vi "Turret_Aim.vi"(6 "Driver Right Thumb":bool, 7 "Left Trigger":dbl, 8 "Orange Limit Pressed":bool, 9 "Blue Limit Pressed":bool, 10 "Right Bumper":bool, 11 "Left Bumper":bool) -> ()   [LabVIEW 2020]
uses:
  <vilib>/Rock Robotics/WPI/ThirdParty/Phoenix-LabVIEW/Motor Controller/Controls/CTRE_Phoenix_MotorControl_ControlMode.ctl
  <vilib>/Rock Robotics/WPI/ThirdParty/Phoenix-LabVIEW/Motor Controller/Get/CTRE_Phoenix_MotorController_IntegratedSensorData_TalonFX.vi
  <vilib>/addons/control/pid/pid.llb/PID (DBL).vi
  <vilib>/Rock Robotics/Network Tables/NT Write Number.vi
  <vilib>/addons/control/pid/NI_PID_pid.lvlib
panel:
  in  "setpoint":dbl=1800.0 format="%#_13g"
  in  "Turret Home":T1={"proportional gain (Kc)"=0.005, "integral time (Ti, min)"=0.0, "derivative time (Td, min)"=2e-05} {"derivative time (Td, min)" format="%.6f"; "integral time (Ti, min)" format="%.3f"; "proportional gain (Kc)" format="%.3f"}
  out "Ty":dbl
  in  "PID gains 5":T1={"proportional gain (Kc)"=-0.015, "integral time (Ti, min)"=0.0, "derivative time (Td, min)"=2e-05} {"derivative time (Td, min)" format="%.6f"; "integral time (Ti, min)" format="%.3f"; "proportional gain (Kc)" format="%.3f"}
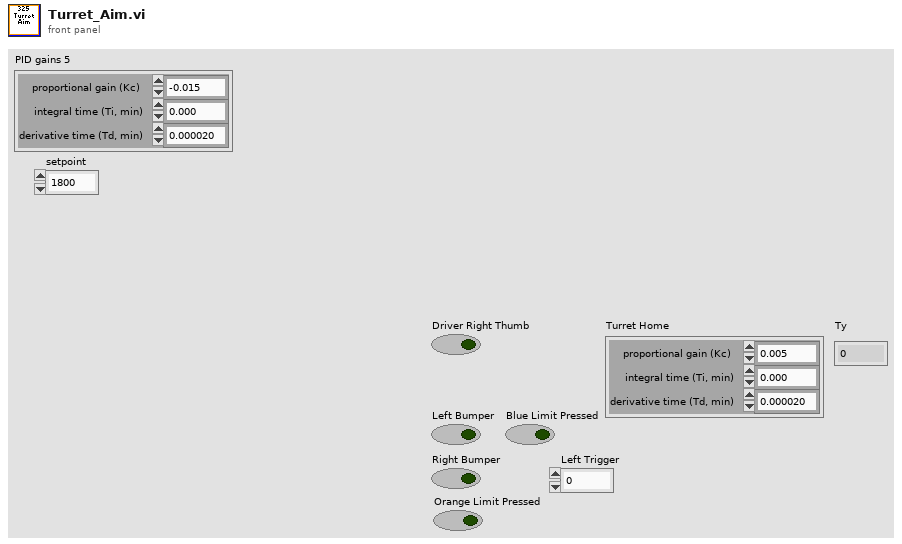
[diagram p1: front panel]
types:
  T1 = cluster{"proportional gain (Kc)":dbl, "integral time (Ti, min)":dbl, "derivative time (Td, min)":dbl}
  T2 = typedef "CTRE_Phoenix_MotorControl_ControlMode.ctl" = u16
  T3 = typedef "WPI_MotorControlDeviceRef.ctl" = cluster{"DeviceStatus":errorcluster, "Type":T4, "PWM":cluster{"PWM Channel":T5, "DeadBand":T6}, "CAN":cluster{"Device Number":u8, "SetOutput VI Ref":variant, "GetOutput VI Ref":variant, "Enable VI Ref":variant, "Disable VI Ref":variant, "Data":variant}, "Invert":bool, "DIO PWM":cluster{"PWM \"Enable\" Channel":T5, "DIOChannel":T7, "PWM Rate":dbl}}
  T4 = typedef "WPI_MotorControlType.ctl" = enum16{"PWM", "CAN", "DIO PWM"}
  T5 = typedef "FPGA_DIOPWMChannel.ctl" = enum8{"PWM 0", "PWM 1", "PWM 2", "PWM 3", "PWM 4", "PWM 5", "PWM 6", "PWM 7", "PWM 8", "PWM 9", "PWM MXP 0", "PWM MXP 1", "PWM MXP 2", "PWM MXP 3", "PWM MXP 4", "PWM MXP 5", "PWM MXP 6", "PWM MXP 7", "PWM MXP 8", "PWM MXP 9", "Invalid"}
  T6 = typedef "WPI_PWMDeadband.ctl" = cluster{"Name":string, "maxPositivePwm":i32, "minPositivePwm":i32, "centerPwm":i32, "maxNegativePwm":i32, "minNegativePwm":i32, "angularRange":u16}
  T7 = typedef "FPGA_DIOChannel.ctl" = enum8{"DIO 0", "DIO 1", "DIO 2", "DIO 3", "DIO 4", "DIO 5", "DIO 6", "DIO 7", "DIO 8", "DIO 9", "DIO MXP 0", "DIO MXP 1", "DIO MXP 2", "DIO MXP 3", "DIO MXP 4", "DIO MXP 5", "DIO MXP 6", "DIO MXP 7", "DIO MXP 8", "DIO MXP 9", "DIO MXP 10", "DIO MXP 11", "DIO MXP 12", "DIO MXP 13", "DIO MXP 14", "DIO MXP 15", "SPI Port CS1", "SPI Port CS2", "SPI Port CS3", "SPI Port MISO", "SPI Port MOSI", "Invalid"}
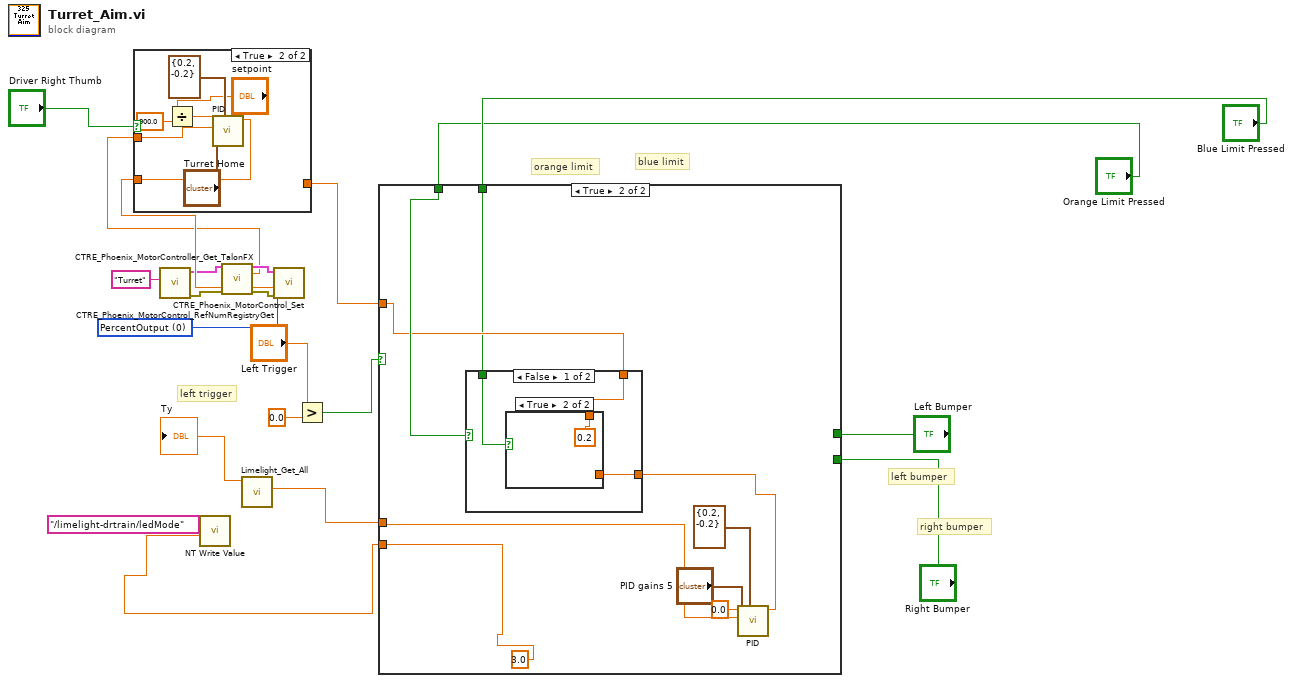
[diagram p0: block diagram]
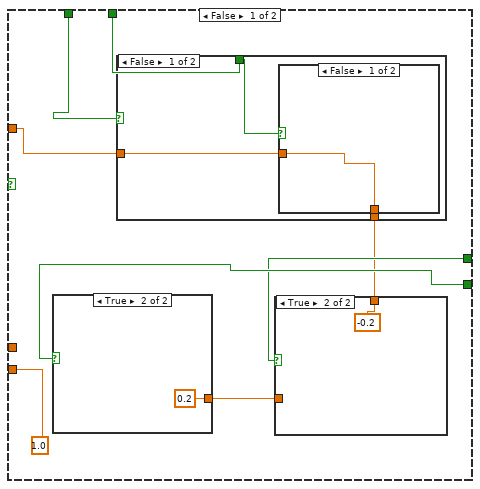
[diagram p3: hidden frame]
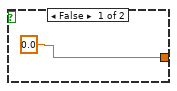
[diagram p5: hidden frame]
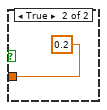
[diagram p6: hidden frame]
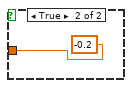
[diagram p7: hidden frame]
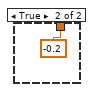
[diagram p9: hidden frame]
diagram:
  w20 = T2 0 items=["PercentOutput"=0, "Position"=1, "Velocity"=2, "Current"=3, "Follower"=5, "MotionProfile"=6, "MotionMagic"=7, "MotionProfileArc"=10, "Disabled"=15] ("Control Mode")
  # "left trigger"
  # "right bumper"
  # "left bumper"
  # "blue limit"
  # "orange limit"
  n1 = call <vilib>:"CTRE_Phoenix_MotorControl_RefNumRegistryGet.vi"("refnum name"="Turret") -> ("error out"=w3:errorcluster, "PhoenixMotorControlDevRef"=w6:T3)  [unwired: 9 in]
  n2 = call-poly <vilib>:"CTRE_Phoenix_MotorController_Get_TalonFX.vi"("PhoenixMotorControlDevRef"=w6, "error in"=w3) -> ("PhoenixMotorControlDevRef"=w5:T3, "Position"=w1:dbl, "error out"=w4:errorcluster)  [unwired: 9 in, 2 out]
  n3 = call "Limelight_Get_All.vi"() -> ("Tx"=w17:dbl, "Ty"=→"Ty":dbl)  [unwired: 10 in]
  n4 = Greater?(x="Left Trigger", y=0.0) -> (0:w18:bool)
  n5 = case shown="True" w18 {
    tunnel: w17 -> [_ w48]
    tunnel: [w23 w43] -> w7
    tunnel: "Orange Limit Pressed" -> [w29 w44]
    tunnel: "Blue Limit Pressed" -> [w28 w41]
    tunnel: "Right Bumper" -> [w27 _]
    tunnel: "Left Bumper" -> [w26 _]
    tunnel: [1.0 ("Numeric") 3.0 ("ledMode")] -> w9
    frame False {
      n6 = case shown="True" w27 {
        tunnel: [0.0 ("output") 0.2 ("output")] -> w25
        frame False {
        }
        frame True {
        }
      }
      n7 = case shown="True" w26 {
        tunnel: w25 -> [w30 _]
        tunnel: [w30 -0.2 ("output")] -> w24
        frame False {
        }
        frame True {
        }
      }
      n8 = case shown="False" w29 {
        tunnel: w28 -> [w36 _]
        tunnel: w24 -> [w35 _]
        tunnel: [w34 -0.2 ("output")] -> w23
        frame False {
          n9 = case shown="False" w36 {
            tunnel: w35 -> [w37 _]
            tunnel: [w37 0.2 ("output")] -> w34
            frame False {
            }
            frame True {
            }
          }
        }
        frame True {
        }
      }
    }
    frame True {
      n10 = call-poly <vilib>:"PID.vi"("output range"=cluster{"output high":dbl, "output low":dbl} {"output high"=0.2, "output low"=-0.2}, "PID gains"="PID gains 5", "process variable"=w48, "setpoint"=0.0) -> ("output"=w42:dbl)  [unwired: 6 in, 1 out]
      n11 = case shown="False" w44 {
        tunnel: [w50 -0.2 ("output")] -> w43
        tunnel: w42 -> [w49 _]
        tunnel: w41 -> [w51 _]
        frame False {
          n12 = case shown="True" w51 {
            tunnel: [w52 0.2 ("output")] -> w50
            tunnel: w49 -> [w52 _]
            frame False {
            }
            frame True {
            }
          }
        }
        frame True {
        }
      }
    }
  }
  n13 = case shown="True" "Driver Right Thumb" {
    tunnel: [w55 w59] -> w8
    tunnel: w7 -> [w55 _]
    tunnel: w1 -> [_ w62]
    frame False {
    }
    frame True {
      n14 = Divide(x="setpoint", y=900.0) -> (x/y=w58:dbl)
      n15 = call-poly <vilib>:"PID.vi"("output range"=cluster{"output high":dbl, "output low":dbl} {"output high"=0.2, "output low"=-0.2}, "PID gains"="Turret Home", "process variable"=w62, "setpoint"=w58) -> ("output"=w59:dbl)  [unwired: 6 in, 1 out]
    }
  }
  n16 = call-poly <vilib>:"NT Write Value.vi"("Numeric"=w9, "Name"="/limelight-drtrain/ledMode") -> ()  [unwired: 9 in, 1 out]
  n17 = call <vilib>:"CTRE_Phoenix_MotorControl_Set.vi"("error in (no error)"=w4, "Output"=w8, "Control Mode"=w20, "PhoenixMotorControlDevRef"=w5) -> ()  [unwired: 6 in, 2 out]
